vi "Get Channels.vi"(7 "GUID (Default Channel)":string="03D3BB99-1485-13A6-561D1F898F032919", 8 "error in (no error)":errorcluster, 11 "Item Ref in":T1 format="%.0x") -> (0 "error out":errorcluster, 2 "Channels refs":T1[](array[typedef]) format="%.0x", 3 "Item Ref out":T1 format="%.0x")   [LabVIEW 2019, in "DSF Shared.lvlib"]
uses:
  DSF Shared.lvlib
  <vilib>/NI VeriStand/Custom Device API/Custom Device Item Ref.ctl
  <vilib>/NI VeriStand/Custom Device API/Custom Device API.lvlib
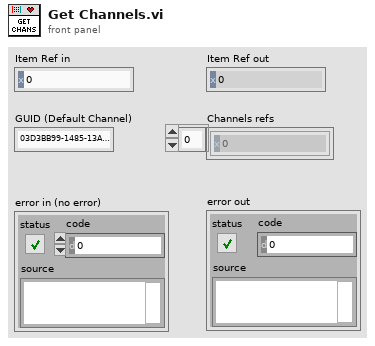
[diagram p1: front panel]
types:
  T1 = typedef "Custom Device API.lvlib/Custom Device Item Ref.ctl" = u64
  T2 = typedef "Custom Device API.lvlib/Custom Device Item Info.ctl" = cluster{"Name":string, "Is Channel":bool, "GUID":string, "Is Waveform":bool}
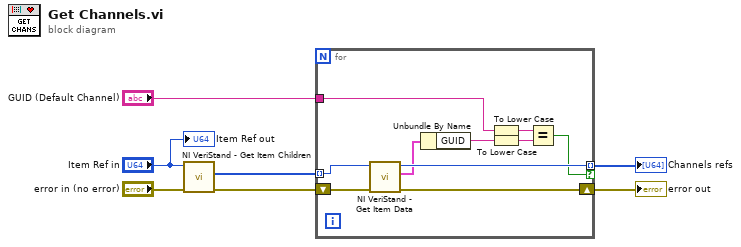
[diagram p0: block diagram]
diagram:
  n1 = call <vilib>:"NI VeriStand - Get Item Children.vi"("error in (no error)"="error in (no error)", "Item Ref in"="Item Ref in") -> ("error out"=w6:errorcluster, "Child Refs"=w4:T1[])  [unwired: 6 in, 2 out]
  n2 = for {
    shift-right: [w16] -> w3
    shift-left: w6 -> [w17]
    tunnel: w4 -> [w15] mode=indexing
    tunnel: [w13] -> w2 mode=indexing if=w12
    tunnel: "GUID (Default Channel)" -> [w10]
    n3 = call <vilib>:"NI VeriStand - Get Item Data.vi"("error in (no error)"=w17, "Item Ref in"=w15) -> ("error out"=w16:errorcluster, "Item Info"=w11:T2, "Item Ref out"=w13:T1)  [unwired: 6 in, 1 out]
    n4 = Unbundle By Name(w11) -> ("GUID"=w14:string)
    n5 = To Lower Case(string=w10) -> (all lower case string=w9:string)
    n6 = To Lower Case(string=w14) -> (all lower case string=w8:string)
    n7 = Equal?(x=w9, y=w8) -> (x = y?=w12:bool)
  }
  "error out" <- w3
  "Channels refs" <- w2
  "Item Ref out" <- "Item Ref in"
